vi "Set Property.vi"(0 "SigMan in":refnum<class "SignalManager.lvclass">, 5 "chan":string, 7 "param":string, 9 "value":dbl, 11 "error in (no error)":errorcluster) -> (4 "SigMan out":refnum<class "SignalManager.lvclass">, 15 "error out":errorcluster)   [LabVIEW 2015, in "SignalManager.lvclass"]
uses:
  SignalManager.lvclass
  SignalManager.lvclass/SignalManager.ctl
  Channel/Channel.lvclass/Channel.ctl
  Channel/Read Name.vi
  Channel/Channel.lvclass
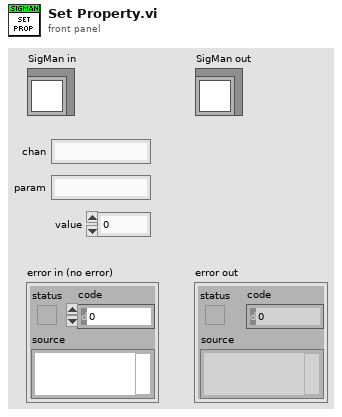
[diagram p1: front panel]
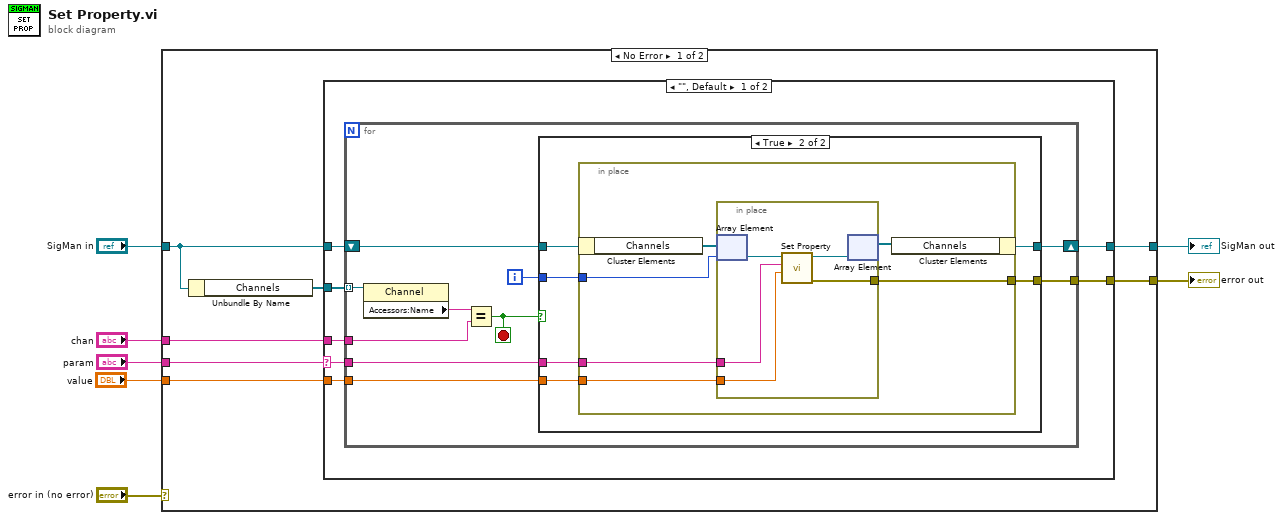
[diagram p0: block diagram]
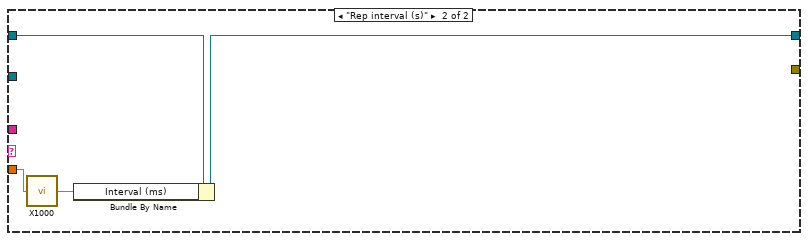
[diagram p3: hidden frame]
diagram:
  n1 = case shown="No Error" "error in (no error)" {
    selector: "error in (no error)" -> [_ w55]
    tunnel: [w8 w55] -> w6
    tunnel: [w9 w54] -> w4
    tunnel: "SigMan in" -> [w10 w54]
    tunnel: "chan" -> [w13 _]
    tunnel: "param" -> [w12 _]
    tunnel: "value" -> [w11 _]
    frame No Error {
      n2 = Unbundle By Name(w10) -> ("Channels"=w14:refnum<class "Channel.lvclass">[])
      n3 = case shown="\"\", Default" w12 {
        selector: w12 -> [w19 _]
        tunnel: w14 -> [w21 _]
        tunnel: w13 -> [w20 _]
        tunnel: w11 -> [w18 w52]
        tunnel: w10 -> [w17 w53]
        tunnel: [w16 w50] -> w9
        tunnel: [w15 _] -> w8
        frame "", Default {
          n4 = for {
            tunnel: w21 -> [w31] mode=indexing
            tunnel: w20 -> [w29]
            tunnel: w19 -> [w24]
            tunnel: w18 -> [w23]
            shift-right: [w26] -> w16
            shift-left: w17 -> [w28]
            tunnel: [w22] -> w15
            i -> [w25]
            stop <- w27 stop-if-true
            n5 = property class="Channel"(reference=w31) -> ("Accessors:Name"=w30:string)  [unwired: 1 in, 2 out]
            n6 = Equal?(x=w30, y=w29) -> (x = y?=w27:bool)
            n7 = case shown="True" w27 {
              tunnel: w28 -> [w32 w38]
              tunnel: [w32 w36] -> w26
              tunnel: w25 -> [_ w37]
              tunnel: w24 -> [_ w35]
              tunnel: w23 -> [_ w34]
              tunnel: [_ w33] -> w22
              frame False {
              }
              frame True {
                n8 = in-place {
                  in-place-border: w37 -> [w43]
                  in-place-border: w35 -> [w41]
                  in-place-border: w34 -> [w40]
                  in-place-border: [w39] -> w33
                  n9 = in-place-cluster #1(w38) -> ("Channels"=w44:refnum<class "Channel.lvclass">[])
                  n10 = in-place {
                    in-place-border: w41 -> [w47]
                    in-place-border: w40 -> [w46]
                    in-place-border: [w45] -> w39
                    n11 = in-place-array #2(w44, w43) -> (w49:refnum<class "Channel.lvclass">)
                    n12 = call "Set Property.vi"("Value"=w46, "Property"=w47, "Channel in"=w49) -> ("error out"=w45:errorcluster, "Channel out"=w48:refnum<class "Channel.lvclass">)  [unwired: 7 in]
                    n13 = in-place-array #2(w48) -> (w42:refnum<class "Channel.lvclass">[])  [unwired: 1 out]
                  }
                  n14 = in-place-cluster #1("Channels"=w42) -> (w36:refnum<class "SignalManager.lvclass">)
                }
              }
            }
          }
        }
        frame "Rep interval (s)" {
          n15 = call "X1000.vi"("X"=w52) -> ("X/1000"=w51:dbl)
          n16 = Bundle By Name(cluster=w53, "Interval (ms)"=w51) -> (w50:refnum<class "SignalManager.lvclass">)
        }
      }
    }
    frame Error {
    }
  }
  "error out" <- w6
  "SigMan out" <- w4
